vi "Check Range.vi"(8 "error in (no error)":errorcluster, 9 "Baratron 2":dbl, 10 "Baratron 1":dbl, 11 "cRIO Vacuum in":refnum<class "cRIO Vacuum.lvclass">) -> (0 "error out":errorcluster, 1 "Baratron 2":dbl, 2 "Baratron 1":dbl, 3 "cRIO Vacuum out":refnum<class "cRIO Vacuum.lvclass">, 4 "B2 out of range":bool)   [LabVIEW 2015, in "cRIO-Carbondioxide.lvlib" / "CO2-Actor.lvlib" / "cRIO Vacuum.lvclass"]
uses:
  cRIO Vacuum.lvclass
  cRIO Vacuum.lvclass/cRIO Vacuum.ctl
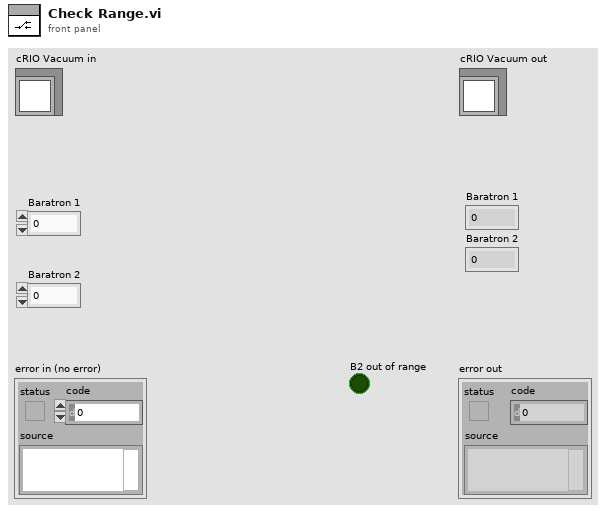
[diagram p1: front panel]
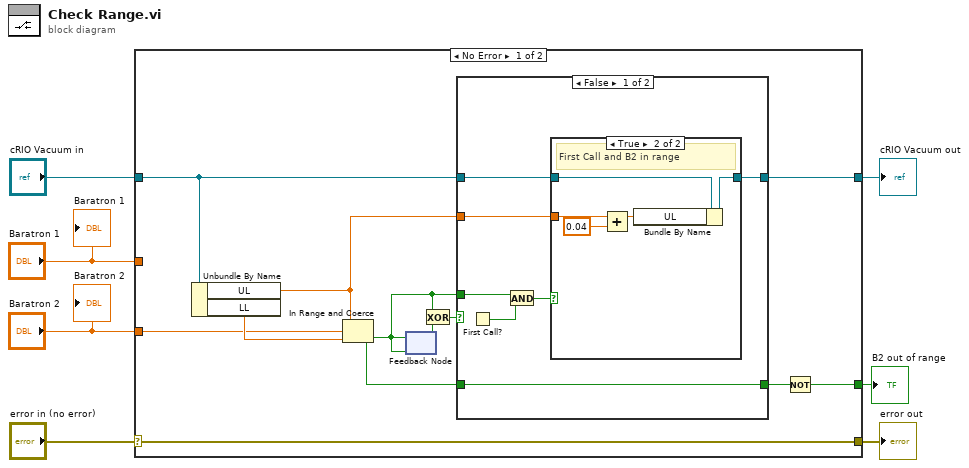
[diagram p0: block diagram]
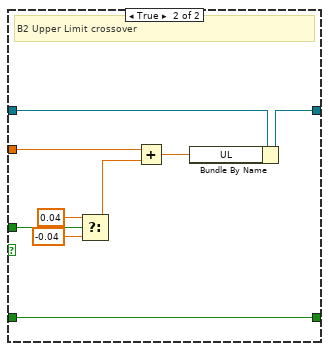
[diagram p3: hidden frame]
diagram:
  n1 = case shown="No Error" "error in (no error)" {
    selector: "error in (no error)" -> [w18 w42]
    tunnel: [w18 w42] -> w6
    tunnel: [w14 w41] -> w4
    tunnel: "cRIO Vacuum in" -> [w17 w41]
    tunnel: "Baratron 1" -> [_ _]
    tunnel: "Baratron 2" -> [w13 _]
    tunnel: [w15 _] -> w3
    frame No Error {
      n2 = Unbundle By Name(w17) -> ("UL"=w9:dbl, "LL"=w16:dbl)
      n3 = In Range and Coerce(upper limit=w9, x=w13, lower limit=w16) -> (In Range?=w8:bool)  [unwired: 1 out]
      n4 = feedback-in #1(w8) -> ()
      n5 = feedback #1(w8) -> (w11:bool)
      n6 = Exclusive Or(1:w11, 2:w8) -> (0:w10:bool)
      n7 = case shown="False" w10 {
        tunnel: w17 -> [w25 w40]
        tunnel: [w21 w39] -> w14
        tunnel: [w24 w38] -> w12
        tunnel: w8 -> [w24 w38]
        tunnel: w9 -> [w19 w34]
        tunnel: w8 -> [w23 w37]
        frame False {
          n8 = First Call?() -> (First Call?: T/F=w22:bool)
          n9 = And(x=w23, y=w22) -> (x .and. y?=w20:bool)
          n10 = case shown="True" w20 {
            tunnel: w25 -> [w26 w31]
            tunnel: [w26 w30] -> w21
            tunnel: w19 -> [_ w29]
            frame False {
            }
            frame True {
              # "First Call and B2 in range"
              n11 = Add(x=w29, y=0.04) -> (x+y=w28:dbl)
              n12 = Bundle By Name(cluster=w31, "UL"=w28) -> (w30:refnum<class "cRIO Vacuum.lvclass">)
            }
          }
        }
        frame True {
          # "B2 Upper Limit crossover"
          n13 = Select(t=0.04, s=w37, f=-0.04) -> (s? t:f=w32:dbl)
          n14 = Add(x=w34, y=w32) -> (x+y=w33:dbl)
          n15 = Bundle By Name(cluster=w40, "UL"=w33) -> (w39:refnum<class "cRIO Vacuum.lvclass">)
        }
      }
      n16 = Not(x=w12) -> (.not. x?=w15:bool)
    }
    frame Error {
    }
  }
  "error out" <- w6
  "cRIO Vacuum out" <- w4
  "B2 out of range" <- w3
  "Baratron 1" <- "Baratron 1"
  "Baratron 2" <- "Baratron 2"
